vi "Load Subitems.vi"(7 "defer fp updates?(T)":bool=TRUE, 8 "error in (no error)":errorcluster, 9 "Tag":string, 11 "Application Data in":T1) -> (0 "error out":errorcluster, 1 "item children":string[](array[string]), 3 "Application Data out":T1)   [LabVIEW 2017, in "DSF Configuration Utility.lvlib"]
uses:
  DSF Configuration Utility.lvlib
  Main VI/Application Data.ctl
  Core/Classes/Configuration/Configuration Session.lvclass
  Main VI/View Mode.ctl
  Create New Tree Item.vi
  Core/Classes/Configuration/Deprecated/Read Settings by ID.vi
  Core/Classes/Configuration/Deprecated/Read Channel by ID.vi.vi
  Core/Classes/Configuration/Deprecated/Remove ID.vi
  Core/Classes/Configuration/Deprecated/Read Transfer by ID.vi
  Core/Classes/Configuration/Deprecated/Read Group by ID.vi.vi
  Core/Classes/Configuration/Deprecated/Read Plugin by ID.vi
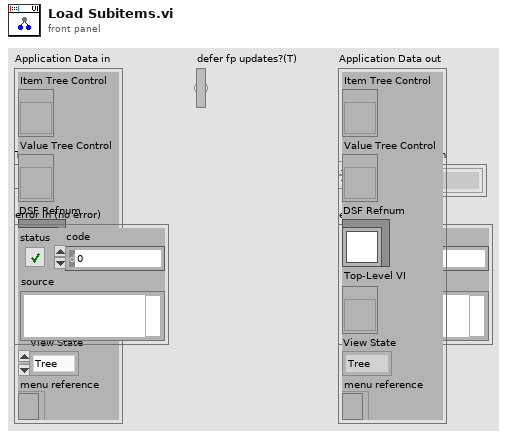
[diagram p1: front panel]
types:
  T1 = typedef "DSF Configuration Utility.lvlib/Application Data.ctl" = cluster{"Item Tree Control":refnum<vi>, "Value Tree Control":refnum<vi>, "DSF Refnum":refnum<class "Configuration Session.lvclass">, "Top-Level VI":refnum<vi>, "View State":T2, "menu reference":refnum<k9>}
  T2 = typedef "DSF Configuration Utility.lvlib/View Mode.ctl" = enum16{"Tree", "List"}
  T3 = typedef "DSF Configuration Utility.lvlib/Tree Item Type.ctl" = enum16{"Plugin", "Group", "Transfer", "Channel", "Setting"}
  T4 = typedef "DSF Core.lvlib/DSF Plugin Info.ctl" = cluster{"components":string[], "timing":T5, "group ids":string[], "settings id":string, "threads":T6[]}
  T5 = typedef "DSF Core.lvlib/DSF Timing Info.ctl" = cluster{"priority":u64, "decimation":u64, "offset":u64}
  T6 = typedef "DSF Core.lvlib/DSF Engine Plugin Thread Configuration.ctl" = cluster{"buffer converter settings":T7, "transceiver settings":T7, "custom settings":T7, "processor":i32, "priority offset":i16}
  T7 = typedef "DSF Core.lvlib/DSF Settings Info.ctl" = cluster{"key":string, "value":string}[]
  T8 = typedef "DSF Configuration Utility.lvlib/Tree Item.ctl" = cluster{"Left Cell String":string, "Child Text":string[], "Child Tag":string, "Glyph Index":i32}
  T9 = typedef "DSF Core.lvlib/DSF Group Info.ctl" = cluster{"direction":T10, "timing":T5, "transfer ids":string[], "settings id":string, "thread":i32, "timeout behavior":T11}
  T10 = typedef "DSF Core.lvlib/DSF Direction.ctl" = enum8{"Tx", "Rx"}
  T11 = typedef "DSF Core.lvlib/DSF Timeout Behavior.ctl" = enum8{"Increment Late Count", "Throw Error"}
  T12 = typedef "DSF Core.lvlib/DSF Transfer Info.ctl" = cluster{"byte order":T13, "channel ids":string[], "settings id":string}
  T13 = typedef "DSF Core.lvlib/DSF Byte Order.ctl" = enum8{"big-endian", "little-endian"}
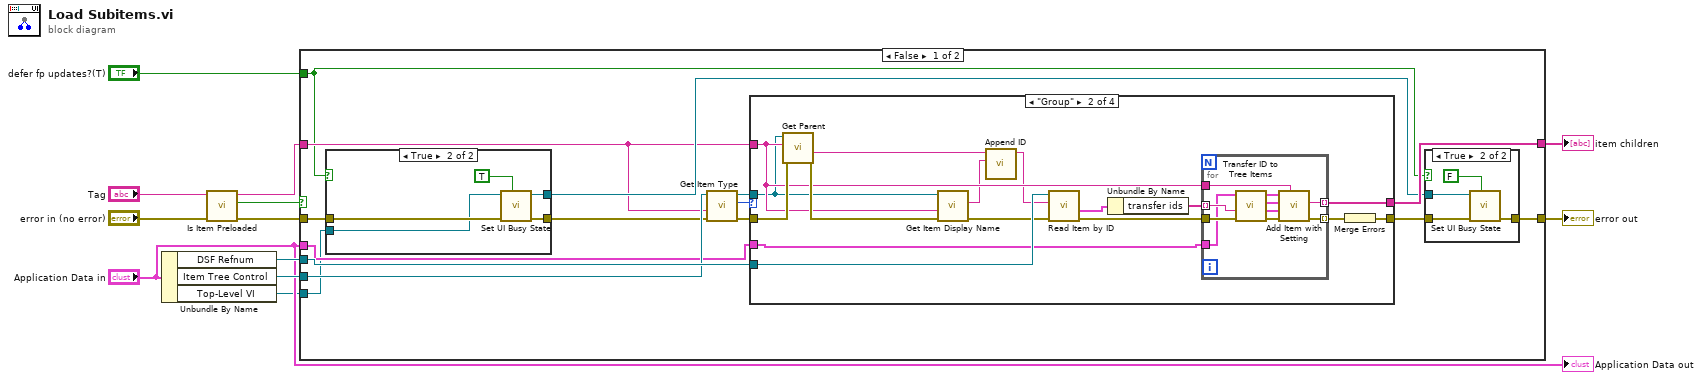
[diagram p0: block diagram]
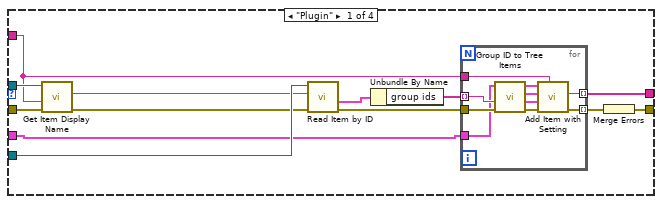
[diagram p4: hidden frame]
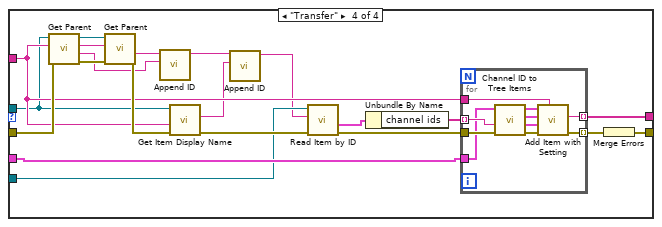
[diagram p6: hidden frame]
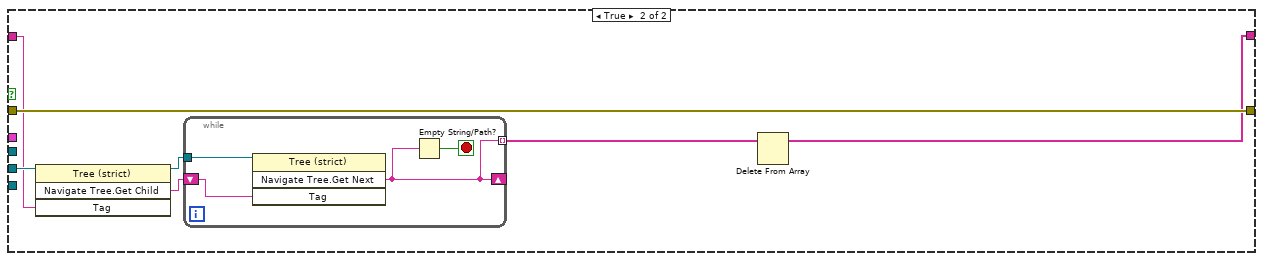
[diagram p7: hidden frame]
diagram:
  n1 = Unbundle By Name("Application Data in") -> ("DSF Refnum"=w5:refnum<class "Configuration Session.lvclass">, "Item Tree Control"=w4:refnum<vi>, "Top-Level VI"=w2:refnum<vi>)
  n2 = call "Is Item Preloaded"("error in (no error)"="error in (no error)", "Tag in"="Tag") -> ("error out"=w9:errorcluster, "replaced"=w11:bool, "Tag out"=w12:string)  [unwired: 7 in]
  n3 = case shown="False" w11 {
    tunnel: w5 -> [w26 _]
    tunnel: w4 -> [w23 w125]
    tunnel: [w16 w126] -> w8
    tunnel: w9 -> [w22 w126]
    tunnel: w12 -> [w14 w124]
    tunnel: [w21 w121] -> w6
    tunnel: "Application Data in" -> [w19 _]
    tunnel: w2 -> [w18 _]
    tunnel: "defer fp updates?(T)" -> [w13 _]
    frame False {
      n4 = case shown="True" w13 {
        tunnel: w22 -> [w33 w38]
        tunnel: w18 -> [_ w37]
        tunnel: [w33 w36] -> w17
        tunnel: [_ w35] -> w15
        frame False {
        }
        frame True {
          n5 = call "Set UI Busy State.vi"("Defer Panel Updates"=TRUE, "error in (no error)"=w38, "VI in"=w37) -> ("error out"=w36:errorcluster, "VI out"=w35:refnum<vi>)  [unwired: 7 in]
        }
      }
      n6 = call "Get Item Type.vi"("error in (no error)"=w17, "Tag"=w14, "TreeControl in"=w23) -> ("error out"=w27:errorcluster, "Item Type"=w25:T3, "TreeControl out"=w20:refnum<vi>)  [unwired: 6 in]
      n7 = case shown="\"Group\"" w25 {
        tunnel: w20 -> [w51 w62 _ w98]
        tunnel: w27 -> [w50 w76 w88 w108]
        tunnel: w26 -> [w49 w75 _ w97]
        tunnel: [w43 w70 w88 w104] -> w24
        tunnel: w14 -> [w40 w66 _ w99]
        tunnel: [w42 w68 _ w101] -> w21
        tunnel: w19 -> [w41 w67 _ w100]
        frame "Plugin" {
          n8 = call "Get Item Display Name.vi"("error in (no error)"=w50, "Tag"=w40, "TreeControl in"=w51) -> ("error out"=w48:errorcluster, "display name"=w39:string)  [unwired: 6 in, 1 out]
          n9 = call-poly "Read Item by ID.vi"("error in (no error)"=w48, "Plugin ID"=w39, "Configuration Session in"=w49) -> ("error out"=w45:errorcluster, "value"=w47:T4)  [unwired: 5 in, 2 out]
          n10 = Unbundle By Name(w47) -> ("group ids"=w46:string[])
          n11 = for {
            tunnel: w46 -> [w61] mode=indexing
            tunnel: w45 -> [w60]
            tunnel: [w58] -> w44 mode=indexing
            tunnel: w40 -> [w53]
            tunnel: [w56] -> w42 mode=indexing
            tunnel: w41 -> [w55]
            n12 = call "Group ID to Tree Items.vi"("error in (no error)"=w60, "Group ID"=w61, "Application Data in"=w55) -> ("error out"=w59:errorcluster, "Settings"=w52:T8, "Item"=w57:T8, "Application Data out"=w54:T1)  [unwired: 5 in]
            n13 = call "Add Item with Setting.vi"("Tag"=w53, "error in (no error)"=w59, "Setting"=w52, "Item"=w57, "Application Data in"=w54) -> ("error out"=w58:errorcluster, "new item tag"=w56:string)  [unwired: 4 in, 1 out]
          }
          n14 = Merge Errors(w44) -> (w43:errorcluster)
        }
        frame "Group" {
          n15 = call "Get Parent.vi"("error in (no error)"=w76, "tag"=w66, "TreeControl in"=w62) -> ("error out"=w77:errorcluster, "parent name"=w65:string)  [unwired: 5 in, 2 out]
          n16 = call "Get Item Display Name.vi"("error in (no error)"=w77, "Tag"=w66, "TreeControl in"=w62) -> ("error out"=w74:errorcluster, "display name"=w64:string)  [unwired: 6 in, 1 out]
          n17 = call "Append ID.vi"("name"=w64, "initial id string (\"\")"=w65) -> ("appended id string"=w63:string)  [unwired: 9 in]
          n18 = call-poly "Read Item by ID.vi"("error in (no error)"=w74, "Group ID"=w63, "Configuration Session in"=w75) -> ("error out"=w71:errorcluster, "value"=w73:T9)  [unwired: 5 in, 2 out]
          n19 = Unbundle By Name(w73) -> ("transfer ids"=w72:string[])
          n20 = for {
            tunnel: w72 -> [w87] mode=indexing
            tunnel: w71 -> [w86]
            tunnel: [w84] -> w69 mode=indexing
            tunnel: w66 -> [w80]
            tunnel: [w83] -> w68 mode=indexing
            tunnel: w67 -> [w81]
            n21 = call "Transfer ID to Tree Items.vi"("error in (no error)"=w86, "Transfer ID"=w87, "Application Data in"=w81) -> ("error out"=w85:errorcluster, "Settings"=w78:T8, "Item"=w79:T8, "Application Data out"=w82:T1)  [unwired: 5 in]
            n22 = call "Add Item with Setting.vi"("Tag"=w80, "error in (no error)"=w85, "Setting"=w78, "Item"=w79, "Application Data in"=w82) -> ("error out"=w84:errorcluster, "new item tag"=w83:string)  [unwired: 4 in, 1 out]
          }
          n23 = Merge Errors(w69) -> (w70:errorcluster)
        }
        frame "Channel", "Setting" {
        }
        frame "Transfer" {
          n24 = call "Get Parent.vi"("error in (no error)"=w108, "tag"=w99, "TreeControl in"=w98) -> ("error out"=w93:errorcluster, "parent name"=w92:string, "parent tag"=w96:string, "TreeControl out"=w89:refnum<vi>)  [unwired: 5 in]
          n25 = call "Get Parent.vi"("error in (no error)"=w93, "tag"=w96, "TreeControl in"=w89) -> ("error out"=w109:errorcluster, "parent name"=w95:string)  [unwired: 5 in, 2 out]
          n26 = call "Append ID.vi"("name"=w92, "initial id string (\"\")"=w95) -> ("appended id string"=w94:string)  [unwired: 9 in]
          n27 = call "Get Item Display Name.vi"("error in (no error)"=w109, "Tag"=w99, "TreeControl in"=w98) -> ("error out"=w107:errorcluster, "display name"=w91:string)  [unwired: 6 in, 1 out]
          n28 = call "Append ID.vi"("name"=w91, "initial id string (\"\")"=w94) -> ("appended id string"=w90:string)  [unwired: 9 in]
          n29 = call-poly "Read Item by ID.vi"("error in (no error)"=w107, "Transfer ID"=w90, "Configuration Session in"=w97) -> ("error out"=w105:errorcluster, "value"=w106:T12)  [unwired: 5 in, 2 out]
          n30 = Unbundle By Name(w106) -> ("channel ids"=w102:string[])
          n31 = for {
            tunnel: w102 -> [w119] mode=indexing
            tunnel: w105 -> [w118]
            tunnel: [w116] -> w103 mode=indexing
            tunnel: w99 -> [w112]
            tunnel: [w115] -> w101 mode=indexing
            tunnel: w100 -> [w114]
            n32 = call "Channel ID to Tree Items.vi"("error in (no error)"=w118, "Channel ID"=w119, "Application Data in"=w114) -> ("error out"=w117:errorcluster, "Settings"=w111:T8, "Item"=w110:T8, "Application Data out"=w113:T1)  [unwired: 5 in]
            n33 = call "Add Item with Setting.vi"("Tag"=w112, "error in (no error)"=w117, "Setting"=w111, "Item"=w110, "Application Data in"=w113) -> ("error out"=w116:errorcluster, "new item tag"=w115:string)  [unwired: 4 in, 1 out]
          }
          n34 = Merge Errors(w103) -> (w104:errorcluster)
        }
      }
      n35 = case shown="True" w13 {
        tunnel: w24 -> [w28 w32]
        tunnel: [w28 w31] -> w16
        tunnel: w15 -> [_ w30]
        frame False {
        }
        frame True {
          n36 = call "Set UI Busy State.vi"("Defer Panel Updates"=FALSE, "error in (no error)"=w32, "VI in"=w30) -> ("error out"=w31:errorcluster)  [unwired: 7 in, 1 out]
        }
      }
    }
    frame True {
      n37 = invoke class="Tree (strict)" method="Navigate Tree.Get Child"(reference=w125, "Tag"=w124) -> (reference out=w123:refnum<vi>, "Navigate Tree:Get Child"=w120:string)  [unwired: 2 in, 2 out]
      n38 = while {
        tunnel: w123 -> [w130]
        tunnel: [w127] -> w122 mode=indexing
        shift-right: [w127] -> _
        shift-left: w120 -> [w128]
        stop <- w129 stop-if-true
        n39 = invoke class="Tree (strict)" method="Navigate Tree.Get Next"(reference=w130, "Tag"=w128) -> ("Navigate Tree:Get Next Item"=w127:string)  [unwired: 2 in, 3 out]
        n40 = Empty String/Path?(string/path=w127) -> (empty?=w129:bool)
      }
      n41 = Delete From Array(array=w122) -> (array with subset deleted=w121:string[])  [unwired: 2 in, 1 out]
    }
  }
  "error out" <- w8
  "item children" <- w6
  "Application Data out" <- "Application Data in"
